vi "SCD - Write err Engineering Data to File.vi"(6 "debug":bool, 8 "error in":errorcluster, 10 "message":string) -> (0 "error out":errorcluster)   [LabVIEW 2014]
doc: "This vi create or open file, which is save in format YYYYMMDD.txt. In this file are logs from CoMP-S Main program."
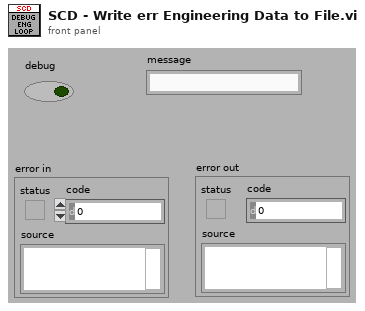
[diagram p1: front panel]
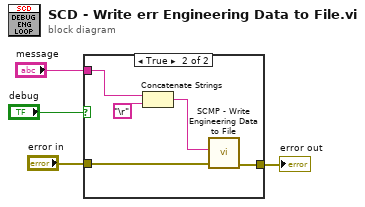
[diagram p0: block diagram]
diagram:
  n1 = case shown="True" "debug" {
    tunnel: "error in" -> [w5 w10]
    tunnel: [w5 w9] -> w2
    tunnel: "message" -> [_ w8]
    frame False {
    }
    frame True {
      n2 = Concatenate Strings(w8, "\r") -> (w6:string)
      n3 = call "SCMP - Write Engineering Data to File.vi"("error in"=w10, "mesage"=w6) -> ("error out"=w9:errorcluster)  [unwired: 6 in, 3 out]
    }
  }
  "error out" <- w2
